vi "XiXi-1(Add DBL，利用同地址结构).vi"(10 "X[-1]":dbl, 11 "Xi":dbl[](array[numeric])) -> (3 "Yi":dbl[](array[numeric]) format="%.2f")   [LabVIEW 2012]
doc: "Calculate sums of consecutive array elements. 0th element of output is equal to x(0)+ x(-1), where x(-1) is an optional scalar input that defaults to zero."
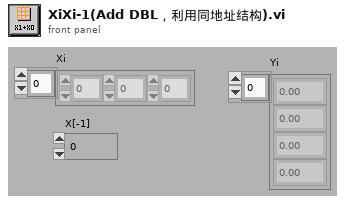
[diagram p1: front panel]
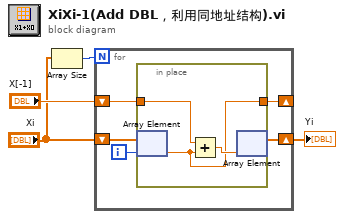
[diagram p0: block diagram]
diagram:
  n1 = Array Size(array="Xi") -> (size(s)=w3:i32)
  n2 = for {
    N: w3 -> [_]
    shift-right: [w7] -> _
    shift-left: "X[-1]" -> [w8]
    shift-right: [w5] -> w1
    shift-left: "Xi" -> [w9]
    i -> [w6]
    n3 = in-place {
      in-place-border: w8 -> [w11]
      in-place-border: [w10] -> w7
      n4 = in-place-array #1(w9, w6) -> (w10:dbl)
      n5 = Add(x=w11, y=w10) -> (x+y=w12:dbl)
      n6 = in-place-array #1(w12) -> (w5:dbl[])  [unwired: 1 out]
    }
  }
  "Yi" <- w1
